vi "ScalingForIR.vi"   [LabVIEW 2012]
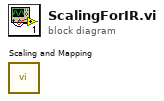
[diagram p0: block diagram]
diagram:
  n1 = call "Scaling and Mapping"() -> ()  [unwired: 10 in, 2 out]
